vi "Get JSON Response Documentation (default).vi"(8 "error in (no error)":errorcluster, 10 "response cluster":variant) -> (0 "error out":errorcluster, 2 "<JSON> Response Documentation":string)   [LabVIEW 2019, in "Instrument.lvlib" / "Help.lvclass"]
uses:
  Help.lvclass
  46988592-c207-47b7-8b61-3fcb2b203627.vi
  <vilib>/JDP Science/JSONtext/Variant to JSON Text.vi
  <vilib>/JDP Science/JSONtext/LVClass Serializer/JSONtext LVClass Serializer.lvclass
  <vilib>/JDP Science/JSONtext/JSONtext.lvlib
  <vilib>/Utility/Data Type/NI_Data Type.lvlib
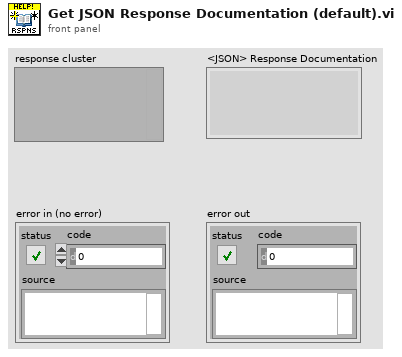
[diagram p1: front panel]
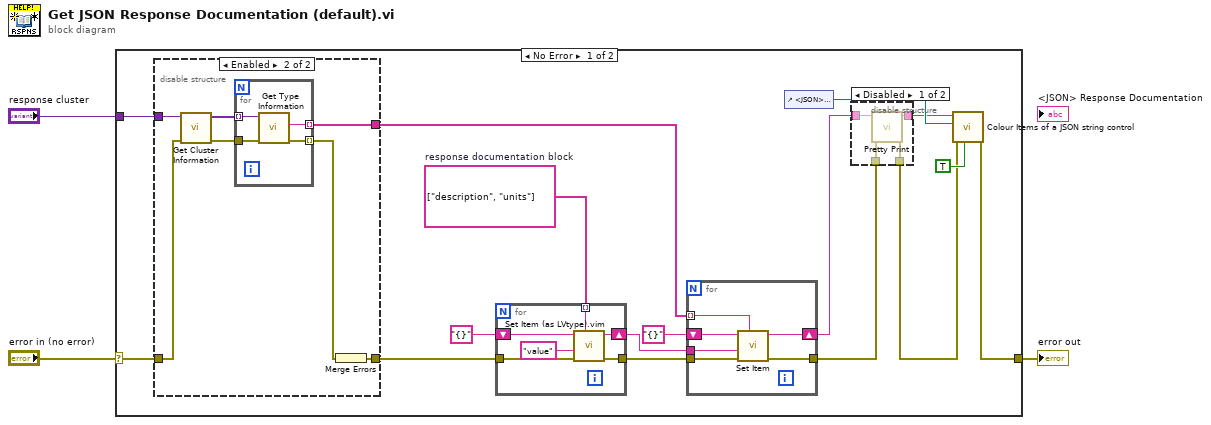
[diagram p0: block diagram]
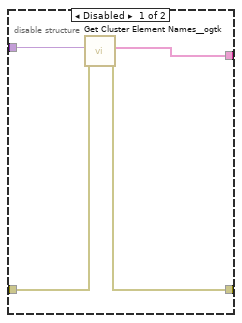
[diagram p2: hidden frame]
diagram:
  n1 = case shown="No Error" "error in (no error)" {
    selector: "error in (no error)" -> [w8 w52]
    tunnel: "response cluster" -> [w7 _]
    tunnel: [w10 w52] -> w1
    frame No Error {
      w16 = string[] ["description", "units"]  # response documentation block
      n2 = disable-structure shown="Enabled" {
        disable-tunnel: w7 -> [w23 w30]
        disable-tunnel: [w22 w28] -> w6
        disable-tunnel: [w21 w24] -> w5
        disable-tunnel: w8 -> [w20 w26]
        frame Disabled {
          n3 = call <userlib>:"Get Cluster Element Names__ogtk.vi"("error in (no error)"=w20, "Cluster"=w23) -> ("error out"=w21:errorcluster, "Element Names"=w22:string[])  [unwired: 8 in]
        }
        frame Enabled {
          n4 = call <vilib>:"Get Cluster Information.vi"("error in (no error)"=w26, "variant"=w30) -> ("error out"=w27:errorcluster, "cluster elements"=w29:variant[])  [unwired: 8 in]
          n5 = for {
            tunnel: w29 -> [w34] mode=indexing
            tunnel: [w33] -> w28 mode=indexing
            tunnel: w27 -> [w32]
            tunnel: [w31] -> w25 mode=indexing
            n6 = call <vilib>:"Get Type Information.vi"("error in (no error)"=w32, "variant"=w34) -> ("error out"=w31:errorcluster, "name"=w33:string)  [unwired: 5 in, 3 out]
          }
          n7 = Merge Errors(w25) -> (w24:errorcluster)
        }
      }
      n8 = for {
        tunnel: w16 -> [w50] mode=indexing
        shift-right: [w49] -> w4
        shift-left: "{}" ("JSON") -> [w51]
        tunnel: [w48] -> w18
        tunnel: w5 -> [w46]
        n9 = call "Set Item (as LVtype).vim"("$Path or Item Name"=w50, "error in (no error)"=w46, "Anything"="value", "JSON"=w51) -> ("error out"=w48:errorcluster, "<JSON>"=w49:string)  [unwired: 4 in, 1 out]
      }
      n10 = for {
        shift-right: [w44] -> w9
        shift-left: "{}" ("JSON") -> [w45]
        tunnel: [w43] -> w11
        tunnel: w4 -> [w42]
        tunnel: w6 -> [w41] mode=indexing
        tunnel: w18 -> [w40]
        n11 = call <vilib>:"Set Item.vi"("$Path or Item Name"=w41, "error in (no error)"=w40, "JSON to Insert"=w42, "JSON"=w45) -> ("error out"=w43:errorcluster, "<JSON>"=w44:string)  [unwired: 4 in, 1 out]
      }
      n12 = control-ref of="<JSON> Response Documentation"() -> (w13:refnum<vi>)
      n13 = disable-structure shown="Disabled" {
        disable-tunnel: [w38 _] -> w14
        disable-tunnel: [w37 w39] -> w12
        disable-tunnel: w11 -> [w36 _]
        disable-tunnel: w9 -> [w35 w39]
        frame Disabled {
          n14 = call <vilib>:"Pretty Print.vi"("error in (no error)"=w36, "JSON"=w35) -> ("error out"=w38:errorcluster, "<JSON>"=w37:string)  [unwired: 7 in, 1 out]
        }
        frame Enabled {
        }
      }
      n15 = call <vilib>:"Colour Items of a JSON string control.vi"("Defer Panel Updates"=TRUE, "error in (no error)"=w14, "String Control"=w13, "JSON"=w12) -> ("error out"=w10:errorcluster)  [unwired: 7 in]
    }
    frame Error {
    }
  }
  "error out" <- w1
